vi "ma_Check Segmented Limit (array segment formula).vi"(0 "Specification Cluster":cluster{"X":dbl[], "Y":string[]}[](array[cluster]) {"X" format="%0.2f"}, 1 "x0":dbl format="%0.2f", 2 "dx":dbl format="%0.2f", 3 "error in":errorcluster) -> (8 "limit spec ok":bool, 9 "1st valid segment index":i32, 10 "error out":errorcluster)   [LabVIEW 2020, in "NI_MAPro.lvlib"]
uses:
  NI_MAPro.lvlib
  NI_MABase.lvlib
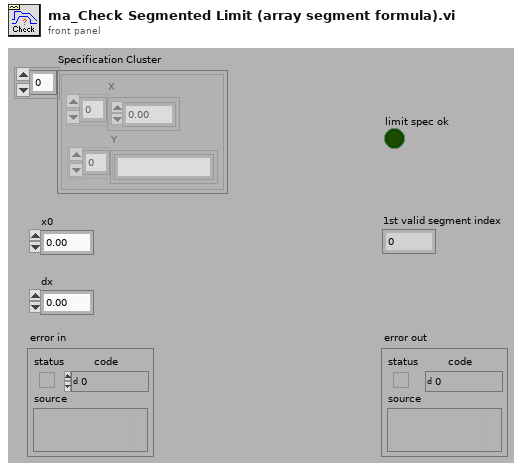
[diagram p1: front panel]
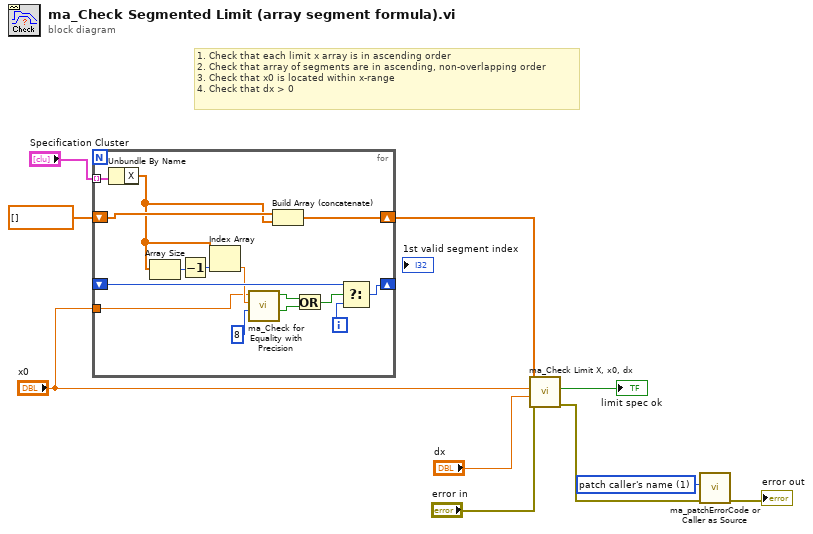
[diagram p0: block diagram]
diagram:
  w7 = u16 1 items=["patch error code", "patch caller's name"] ("operation")
  # "1. Check that each limit x array is in ascending order\n2. Check that array of segments are in ascending, non-overlapping order\n3. Check that x0 is located within x-range\n4. Check that dx > 0"
  n1 = for {
    tunnel: "Specification Cluster" -> [w25] mode=indexing
    shift-right: [w12] -> w1
    shift-left: dbl[] [] -> [w24]
    shift-right: [w20] -> _
    shift-left: _ -> [w21]
    tunnel: "x0" -> [w11]
    i -> [w18]
    n2 = Unbundle By Name(w25) -> ("X"=w19:dbl[])
    n3 = Array Size(array=w19) -> (size(s)=w23:i32)
    n4 = Decrement(x=w23) -> (x-1=w22:i32)
    n5 = Index Array(array=w19, index=w22) -> (element=w17:dbl)
    n6 = call "ma_Check for Equality with Precision.vi"("precision"=8, "n2"=w17, "n1"=w11) -> ("n1 < n2?"=w14:bool, "equal (within precision)"=w15:bool)  [unwired: 7 out]
    n7 = Build Array (concatenate)(w24, w19) -> (w12:dbl[])
    n8 = Or(x=w15, y=w14) -> (x .or. y?=w13:bool)
    n9 = Select(t=w21, s=w13, f=w18) -> (s? t:f=w20:i32)
  }
  n10 = call "ma_Check Limit X, x0, dx.vi"("X"=w1, "x0"="x0", "dx"="dx", "error in"="error in") -> ("limit spec ok"=→"limit spec ok":bool, "error out"=w6:errorcluster)  [unwired: 5 out]
  n11 = call "ma_patchErrorCode or Caller as Source.vi"("error in (no error)"=w6, "operation"=w7) -> ("error out"=→"error out":errorcluster)  [unwired: 2 in, 7 out]
